vi "S2C_ExeScriptDisableStep.vi"(8 "Error In":errorcluster, 11 "Action":string) -> (0 "Error Out":errorcluster)   [LabVIEW 2015]
doc: "Pauses the executable script execution."
uses:
  Globals/S2C_Globals.vi
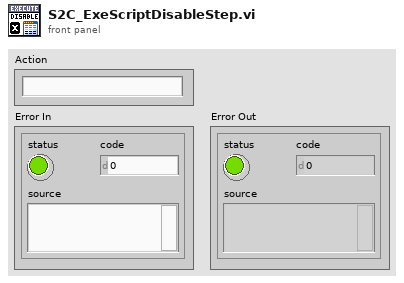
[diagram p1: front panel]
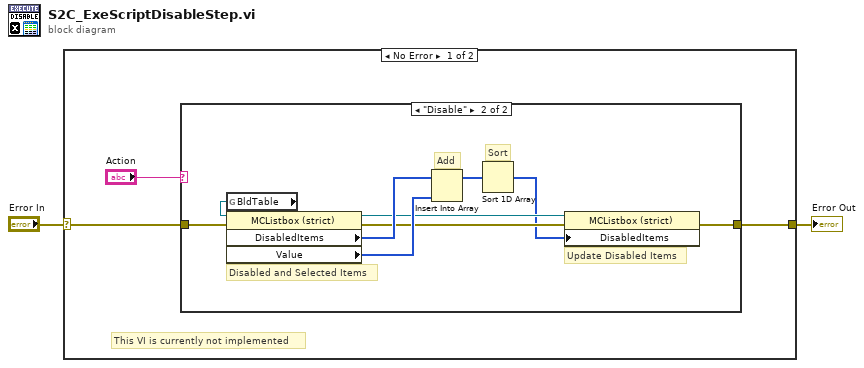
[diagram p0: block diagram]
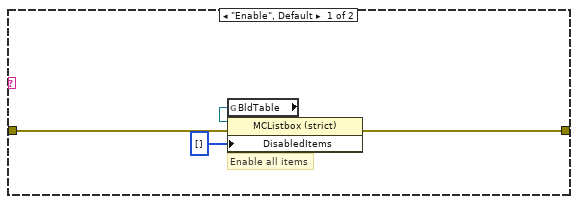
[diagram p2: hidden frame]
diagram:
  n1 = case shown="No Error" "Error In" {
    selector: "Error In" -> [w5 w19]
    tunnel: [w4 w19] -> w1
    frame No Error {
      # "This VI is currently not implemented"
      n2 = case shown="\"Disable\"" "Action" {
        tunnel: w5 -> [w9 w18]
        tunnel: [w7 w10] -> w4
        frame "Enable", Default {
          # "Enable all items"
          n3 = global read "S2C_Globals.vi" "BldTable"() -> (w8:refnum<vi>)
          n4 = property class="MCListbox (strict)"(reference=w8, error in=w9, "DisabledItems"=i32[] [] ("Disabled Items")) -> (error out=w7:errorcluster)  [unwired: 1 out]
        }
        frame "Disable" {
          # "Sort"
          # "Add"
          # "Update Disabled Items"
          # "Disabled and Selected Items"
          n5 = global read "S2C_Globals.vi" "BldTable"() -> (w17:refnum<vi>)
          n6 = property class="MCListbox (strict)"(reference=w17, error in=w18) -> (reference out=w12:refnum<vi>, error out=w13:errorcluster, "DisabledItems"=w15:i32[], "Value"=w14:i32[])
          n7 = Insert Into Array(array=w15, new element=w14) -> (w16:i32[])  [unwired: 1 in]
          n8 = Sort 1D Array(array=w16) -> (sorted array=w11:i32[])
          n9 = property class="MCListbox (strict)"(reference=w12, error in=w13, "DisabledItems"=w11) -> (error out=w10:errorcluster)  [unwired: 1 out]
        }
      }
    }
    frame Error {
    }
  }
  "Error Out" <- w1
